vi "ArmIncrementXYZ.vi"(9 "AddZ":dbl, 10 "AddY":dbl, 11 "AddX":dbl) -> ()   [LabVIEW 2020]
doc: "Increment X,Y,Z values\n\nInput:\n--AddX--Double--how much to increment X\n--AddY--Double--how much to increment Y\n--AddZ--Double--how much to increment Z"
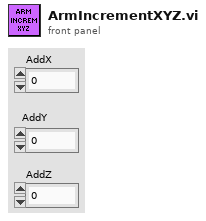
[diagram p1: front panel]
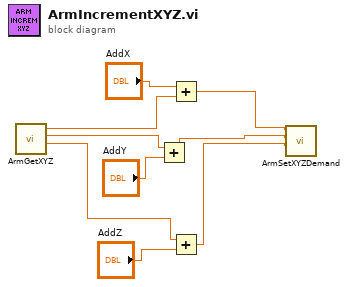
[diagram p0: block diagram]
diagram:
  n1 = call "ArmGetXYZ.vi"() -> ("GetZ"=w4:dbl, "GetY"=w7:dbl, "GetX"=w8:dbl)  [unwired: 9 in]
  n2 = Add(x=w7, y="AddY") -> (x+y=w2:dbl)
  n3 = Add(x="AddX", y=w8) -> (x+y=w3:dbl)
  n4 = Add(x=w4, y="AddZ") -> (x+y=w1:dbl)
  n5 = call "ArmSetXYZDemand.vi"("SetZ"=w1, "SetY"=w2, "SetX"=w3) -> ()  [unwired: 9 in]
